vi "dfd_Synthesis Bank Build Output Waveform.vi"(7 "factor":i32, 8 "error in (no error)":errorcluster, 10 "y1":dbl[](array[numeric]), 11 "subband channel":waveform(dbl)={"t0"=timestamp(0 s since 1904-01-01), "dt"=0.0, "Y"=[]}) -> (0 "error out":errorcluster, 3 "synthesis output":waveform(dbl))   [LabVIEW 2017, in "NI_DigFilter_FilterBank.lvlib"]
uses:
  <vilib>/addons/Digital Filter Design/NI_DigFilter_FilterBank.lvlib
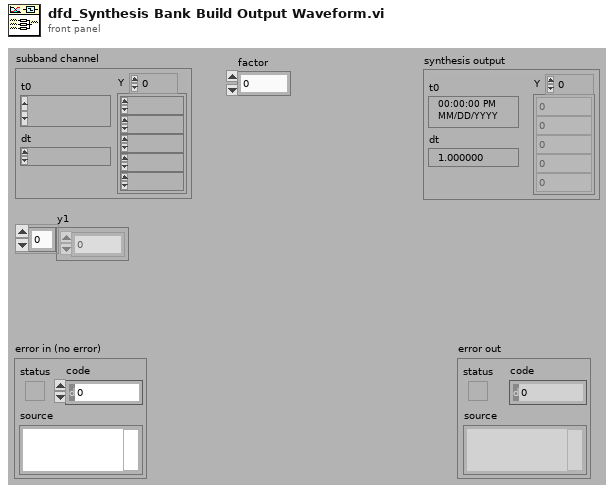
[diagram p1: front panel]
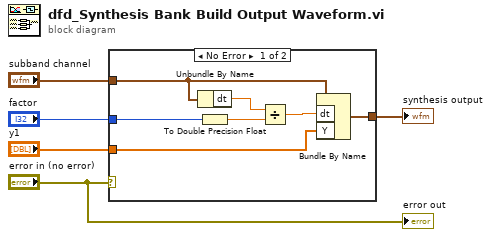
[diagram p0: block diagram]
diagram:
  n1 = case shown="No Error" "error in (no error)" {
    tunnel: [w11 _] -> w5
    tunnel: "y1" -> [w9 _]
    tunnel: "factor" -> [w7 _]
    tunnel: "subband channel" -> [w6 _]
    frame No Error {
      n2 = Unbundle By Name(w6) -> ("dt"=w12:dbl)
      n3 = To Double Precision Float(number=w7) -> (double precision float=w8:dbl)
      n4 = Divide(x=w12, y=w8) -> (x/y=w10:dbl)
      n5 = Bundle By Name(cluster=w6, "dt"=w10, "Y"=w9) -> (w11:waveform(dbl))
    }
    frame Error {
    }
  }
  "synthesis output" <- w5
  "error out" <- "error in (no error)"
